vi "FPGA Read Indicator Scalar Address by Index.vi"(8 "error in (no error)":errorcluster, 9 "index":i32, 10 "Data Type":T1, 11 "FPGA Interface Base in":refnum<class "FPGA Interface Base.lvclass">) -> (0 "error out":errorcluster, 1 "Found?":bool, 2 "Address":u32, 3 "FPGA Interface Base out":refnum<class "FPGA Interface Base.lvclass">)   [LabVIEW 2010, in "FPGA Interface Base.lvclass"]
uses:
  <userlib>/_FPGA Interface Advanced Tools/FPGA Interface Base/FPGA Interface Base.lvclass
  <vilib>/rvi/DataTransferAndStorage/Container/Common/niFpgaDataTypeControl.ctl
  <userlib>/_FPGA Interface Advanced Tools/FPGA Interface Base/FPGA Interface Base.lvclass/FPGA Interface Base.ctl
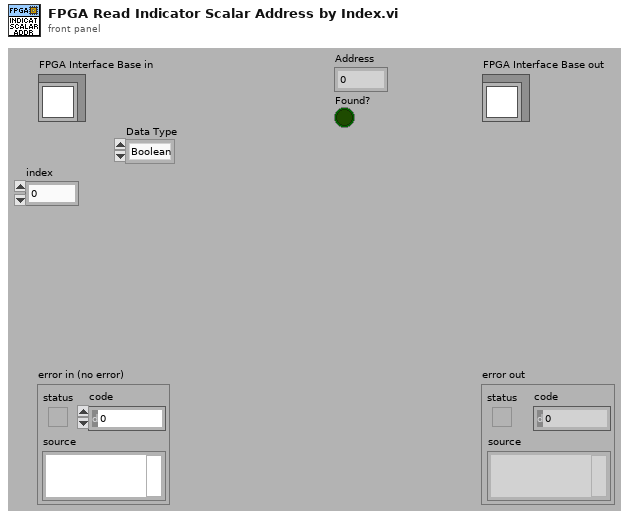
[diagram p1: front panel]
types:
  T1 = typedef "niFpgaDataTypeControl.ctl" = enum32{"Boolean", "I8", "I16", "I32", "I64", "U8", "U16", "U32", "U64", "FXP", "CustomControl"}
  T2 = typedef "FPGA Interface Base.lvclass/FPGA Session.ctl" = refnum<data-value>
  T3 = typedef "FPGA Interface Base.lvclass/FPGA Session Data.ctl" = cluster{"Session Out":u32, "Indicator Scalars":T4, "Indicator Arrays":T6, "Control Scalars":T4, "Control Arrays":T6, "TargetToHost FIFO Channels":T8, "HostToTarget FIFO Channels":T8, "All FIFOs":T9[], "IRQ Context Queue":refnum<queue>}
  T4 = typedef "FPGA Bitfile Utility.lvlib/Scalar Register Set.ctl" = cluster{"Boolean":T5[], "I8":T5[], "I16":T5[], "I32":T5[], "I64":T5[], "U8":T5[], "U16":T5[], "U32":T5[], "U64":T5[]}
  T5 = typedef "FPGA Bitfile Utility.lvlib/Scalar Register.ctl" = cluster{"Address":u32, "Name":string}
  T6 = typedef "FPGA Bitfile Utility.lvlib/Array Register Set.ctl" = cluster{"Boolean":T7[], "I8":T7[], "I16":T7[], "I32":T7[], "I64":T7[], "U8":T7[], "U16":T7[], "U32":T7[], "U64":T7[]}
  T7 = typedef "FPGA Bitfile Utility.lvlib/Array Register.ctl" = cluster{"Address":u32, "Num Elements":u32, "Name":string}
  T8 = typedef "FPGA Bitfile Utility.lvlib/FIFO Channel Set.ctl" = cluster{"Boolean":T9[], "I8":T9[], "I16":T9[], "I32":T9[], "I64":T9[], "U8":T9[], "U16":T9[], "U32":T9[], "U64":T9[]}
  T9 = typedef "FPGA Bitfile Utility.lvlib/FIFO Channel.ctl" = cluster{"Physical Channel":u32, "Name":string}
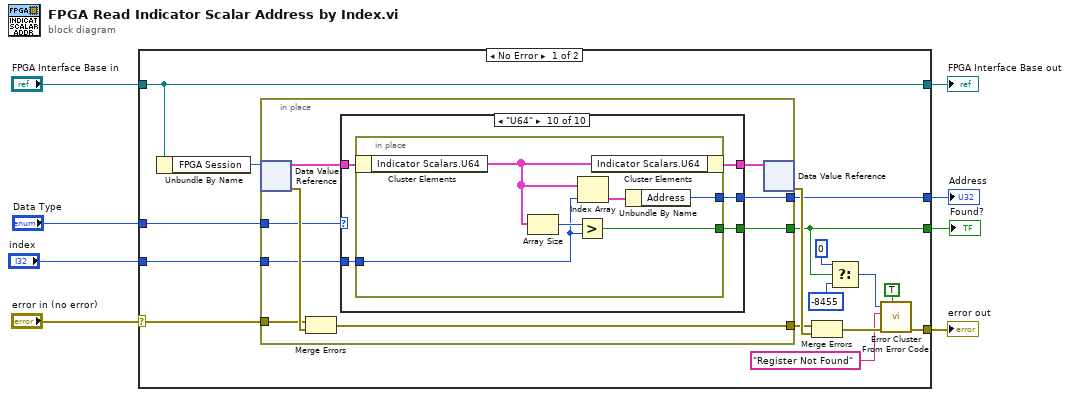
[diagram p0: block diagram]
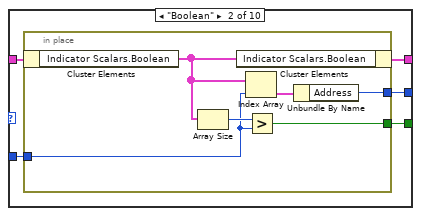
[diagram p3: hidden frame]
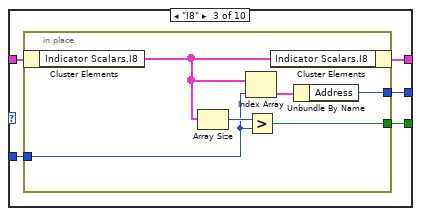
[diagram p4: hidden frame]
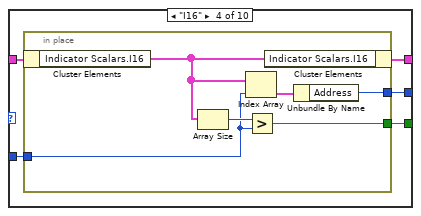
[diagram p5: hidden frame]
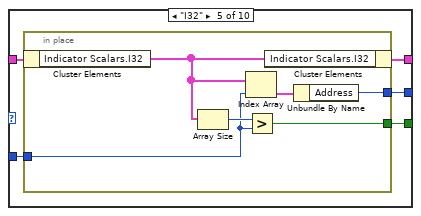
[diagram p6: hidden frame]
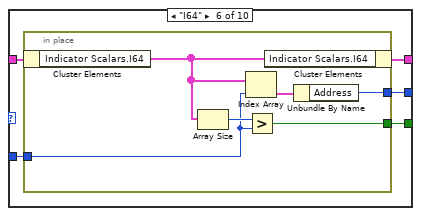
[diagram p7: hidden frame]
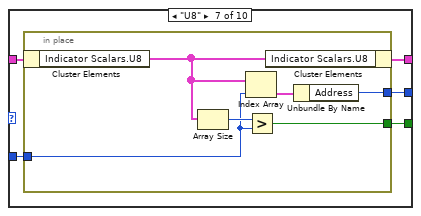
[diagram p8: hidden frame]
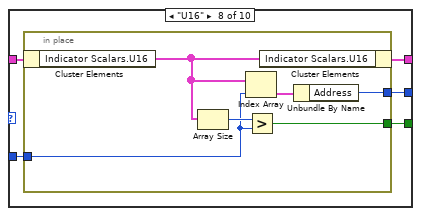
[diagram p9: hidden frame]
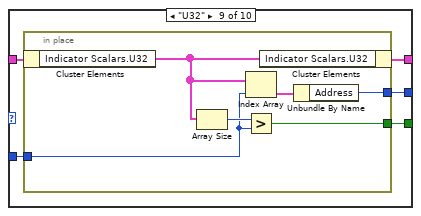
[diagram p10: hidden frame]
diagram:
  n1 = case shown="No Error" "error in (no error)" {
    selector: "error in (no error)" -> [w17 w133]
    tunnel: [w19 w133] -> w7
    tunnel: [w23 w134] -> w5
    tunnel: "FPGA Interface Base in" -> [w23 w134]
    tunnel: [w18 _] -> w4
    tunnel: [w9 _] -> w3
    tunnel: "Data Type" -> [w16 _]
    tunnel: "index" -> [w11 _]
    frame No Error {
      n2 = Unbundle By Name(w23) -> ("FPGA Session"=w20:T2)
      n3 = in-place {
        in-place-border: [w29] -> w18
        in-place-border: [w28] -> w9
        in-place-border: [w27] -> w21
        in-place-border: w17 -> [w26]
        in-place-border: w16 -> [w25]
        in-place-border: w11 -> [w24]
        n4 = in-place-dvr #1(w20) -> (w31:T3, w32:errorcluster)
        n5 = Merge Errors(w26, w32) -> (w27:errorcluster)
        n6 = case shown="\"U64\"" w25 {
          tunnel: w31 -> [w33 w38 w49 w60 w71 w82 w93 w104 w115 w126]
          tunnel: [w33 w37 w48 w59 w70 w81 w92 w103 w114 w125] -> w30
          tunnel: [_ w36 w47 w58 w69 w80 w91 w102 w113 w124] -> w29
          tunnel: [_ w35 w46 w57 w68 w79 w90 w101 w112 w123] -> w28
          tunnel: w24 -> [_ w34 w45 w56 w67 w78 w89 w100 w111 w122]
          frame Default {
          }
          frame "Boolean" {
            n7 = in-place {
              in-place-border: [w44] -> w36
              in-place-border: [w42] -> w35
              in-place-border: w34 -> [w39]
              n8 = in-place-cluster #2(w38) -> ("Indicator Scalars.Boolean"=w41:T5[])
              n9 = Array Size(array=w41) -> (size(s)=w43:i32)
              n10 = in-place-cluster #2("Indicator Scalars.Boolean"=w41) -> (w37:T3)
              n11 = Index Array(array=w41, index=w39) -> (element=w40:T5)
              n12 = Greater?(x=w43, y=w39) -> (0:w42:bool)
              n13 = Unbundle By Name(w40) -> ("Address"=w44:u32)
            }
          }
          frame "I8" {
            n14 = in-place {
              in-place-border: [w55] -> w47
              in-place-border: [w53] -> w46
              in-place-border: w45 -> [w50]
              n15 = in-place-cluster #3(w49) -> ("Indicator Scalars.I8"=w52:T5[])
              n16 = Array Size(array=w52) -> (size(s)=w54:i32)
              n17 = Index Array(array=w52, index=w50) -> (element=w51:T5)
              n18 = Greater?(x=w54, y=w50) -> (0:w53:bool)
              n19 = in-place-cluster #3("Indicator Scalars.I8"=w52) -> (w48:T3)
              n20 = Unbundle By Name(w51) -> ("Address"=w55:u32)
            }
          }
          frame "I16" {
            n21 = in-place {
              in-place-border: [w66] -> w58
              in-place-border: [w64] -> w57
              in-place-border: w56 -> [w61]
              n22 = in-place-cluster #4(w60) -> ("Indicator Scalars.I16"=w63:T5[])
              n23 = Array Size(array=w63) -> (size(s)=w65:i32)
              n24 = Index Array(array=w63, index=w61) -> (element=w62:T5)
              n25 = Greater?(x=w65, y=w61) -> (0:w64:bool)
              n26 = in-place-cluster #4("Indicator Scalars.I16"=w63) -> (w59:T3)
              n27 = Unbundle By Name(w62) -> ("Address"=w66:u32)
            }
          }
          frame "I32" {
            n28 = in-place {
              in-place-border: [w77] -> w69
              in-place-border: [w75] -> w68
              in-place-border: w67 -> [w72]
              n29 = in-place-cluster #5(w71) -> ("Indicator Scalars.I32"=w74:T5[])
              n30 = Array Size(array=w74) -> (size(s)=w76:i32)
              n31 = Index Array(array=w74, index=w72) -> (element=w73:T5)
              n32 = Greater?(x=w76, y=w72) -> (0:w75:bool)
              n33 = in-place-cluster #5("Indicator Scalars.I32"=w74) -> (w70:T3)
              n34 = Unbundle By Name(w73) -> ("Address"=w77:u32)
            }
          }
          frame "I64" {
            n35 = in-place {
              in-place-border: [w88] -> w80
              in-place-border: [w86] -> w79
              in-place-border: w78 -> [w83]
              n36 = in-place-cluster #6(w82) -> ("Indicator Scalars.I64"=w85:T5[])
              n37 = Array Size(array=w85) -> (size(s)=w87:i32)
              n38 = Index Array(array=w85, index=w83) -> (element=w84:T5)
              n39 = Greater?(x=w87, y=w83) -> (0:w86:bool)
              n40 = in-place-cluster #6("Indicator Scalars.I64"=w85) -> (w81:T3)
              n41 = Unbundle By Name(w84) -> ("Address"=w88:u32)
            }
          }
          frame "U8" {
            n42 = in-place {
              in-place-border: [w99] -> w91
              in-place-border: [w97] -> w90
              in-place-border: w89 -> [w94]
              n43 = in-place-cluster #7(w93) -> ("Indicator Scalars.U8"=w96:T5[])
              n44 = Array Size(array=w96) -> (size(s)=w98:i32)
              n45 = Index Array(array=w96, index=w94) -> (element=w95:T5)
              n46 = Greater?(x=w98, y=w94) -> (0:w97:bool)
              n47 = in-place-cluster #7("Indicator Scalars.U8"=w96) -> (w92:T3)
              n48 = Unbundle By Name(w95) -> ("Address"=w99:u32)
            }
          }
          frame "U16" {
            n49 = in-place {
              in-place-border: [w110] -> w102
              in-place-border: [w108] -> w101
              in-place-border: w100 -> [w105]
              n50 = in-place-cluster #8(w104) -> ("Indicator Scalars.U16"=w107:T5[])
              n51 = Array Size(array=w107) -> (size(s)=w109:i32)
              n52 = Index Array(array=w107, index=w105) -> (element=w106:T5)
              n53 = Greater?(x=w109, y=w105) -> (0:w108:bool)
              n54 = in-place-cluster #8("Indicator Scalars.U16"=w107) -> (w103:T3)
              n55 = Unbundle By Name(w106) -> ("Address"=w110:u32)
            }
          }
          frame "U32" {
            n56 = in-place {
              in-place-border: [w121] -> w113
              in-place-border: [w119] -> w112
              in-place-border: w111 -> [w116]
              n57 = in-place-cluster #9(w115) -> ("Indicator Scalars.U32"=w118:T5[])
              n58 = Array Size(array=w118) -> (size(s)=w120:i32)
              n59 = Index Array(array=w118, index=w116) -> (element=w117:T5)
              n60 = Greater?(x=w120, y=w116) -> (0:w119:bool)
              n61 = in-place-cluster #9("Indicator Scalars.U32"=w118) -> (w114:T3)
              n62 = Unbundle By Name(w117) -> ("Address"=w121:u32)
            }
          }
          frame "U64" {
            n63 = in-place {
              in-place-border: [w132] -> w124
              in-place-border: [w130] -> w123
              in-place-border: w122 -> [w127]
              n64 = in-place-cluster #10(w126) -> ("Indicator Scalars.U64"=w129:T5[])
              n65 = Array Size(array=w129) -> (size(s)=w131:i32)
              n66 = Greater?(x=w131, y=w127) -> (0:w130:bool)
              n67 = Index Array(array=w129, index=w127) -> (element=w128:T5)
              n68 = in-place-cluster #10("Indicator Scalars.U64"=w129) -> (w125:T3)
              n69 = Unbundle By Name(w128) -> ("Address"=w132:u32)
            }
          }
        }
        n70 = in-place-dvr #1(w30) -> (w22:errorcluster)  [unwired: 1 out]
      }
      n71 = Merge Errors(w21, w22) -> (w19:errorcluster)
      n72 = Select(t=0, s=w9, f=-8455 ("error code (0)")) -> (s? t:f=w12:i32)
      n73 = call <vilib>:"Error Cluster From Error Code.vi"("show call chain? (False)"=TRUE, "error message (\"\")"="Register Not Found" ("string"), "error code (0)"=w12) -> ()  [unwired: 6 in, 1 out]
    }
    frame Error {
    }
  }
  "error out" <- w7
  "FPGA Interface Base out" <- w5
  "Address" <- w4
  "Found?" <- w3
